vi "Agilent34401AData.vi"(1 "Enum":T1, 3 "Cluster":T2) -> (17 "Cluster 2":T2, 19 "error out":errorcluster)   [LabVIEW 2014]
uses:
  Agilent34401AData.ctl
  FGV.ctl
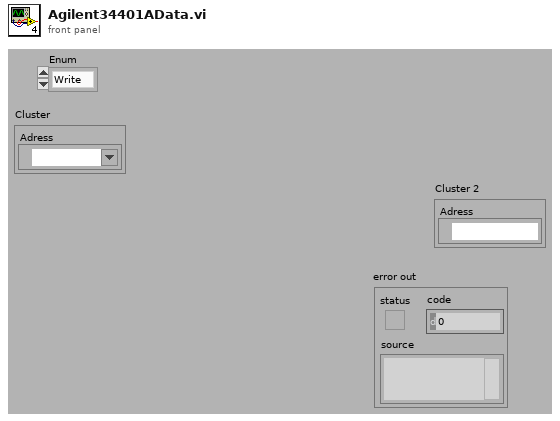
[diagram p1: front panel]
types:
  T1 = typedef "FGV.ctl" = enum16{"Write", "Read", "Init"}
  T2 = typedef "Agilent34401AData.ctl" = cluster{"Adress":refnum<visa-resource-name>}
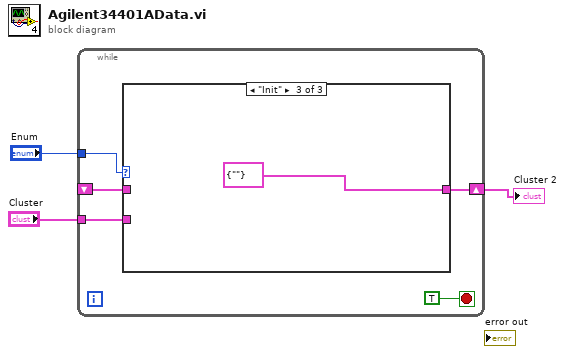
[diagram p0: block diagram]
diagram:
  n1 = while {
    tunnel: "Enum" -> [w7]
    tunnel: "Cluster" -> [w6]
    shift-right: [w4] -> w1
    shift-left: _ -> [w5]
    stop <- TRUE stop-if-true
    n2 = case shown="\"Init\"" w7 {
      tunnel: w6 -> [w9 _ _]
      tunnel: w5 -> [_ w10 _]
      tunnel: [w9 w10 T2 {"Adress"=""} ("Cluster")] -> w4
      frame "Write", Default {
      }
      frame "Read" {
      }
      frame "Init" {
      }
    }
  }
  "Cluster 2" <- w1
